vi "SEM_AMPL_RESULT.vi"(0 "Session In":refnum<visa-resource-name>="TCPIP0::K-N90X0A-00005.local::inst0::INSTR", 11 "error in":errorcluster {"code" format="%.0x"}) -> (1 "ref_freq/ref pwr":dbl[](array[numeric]), 2 "AMPL(DBC)":dbl[](array[numeric]), 3 "SPEC (DBC)":dbl[](array[numeric]), 4 "Session Out":refnum<visa-resource-name>, 15 "error out":errorcluster {"code" format="%.0x"})   [LabVIEW 2018]
doc: "Launches the Instrument I/O Assistant, which you can use to communicate with message-based instruments and graphically parse the response. For example you can communicate with an instrument that uses a serial, Ethernet, or GPIB interface."
panel:
  out "x-y":dbl
  out "Level (dBm)":dbl[](array[numeric]) format="%#.2g"
  out "LIMIT (DBC)":dbl[](array[numeric]) format="%#.2g"
  out "Margin":dbl[](array[numeric]) format="%#.2g"
  out "CA_REF_PWR":dbl
  out "CA_REF_FREQ":dbl
  out "FREQ":dbl[](array[numeric])
  in  "Timeout":u32=3000
  out "array":dbl[](array[numeric])
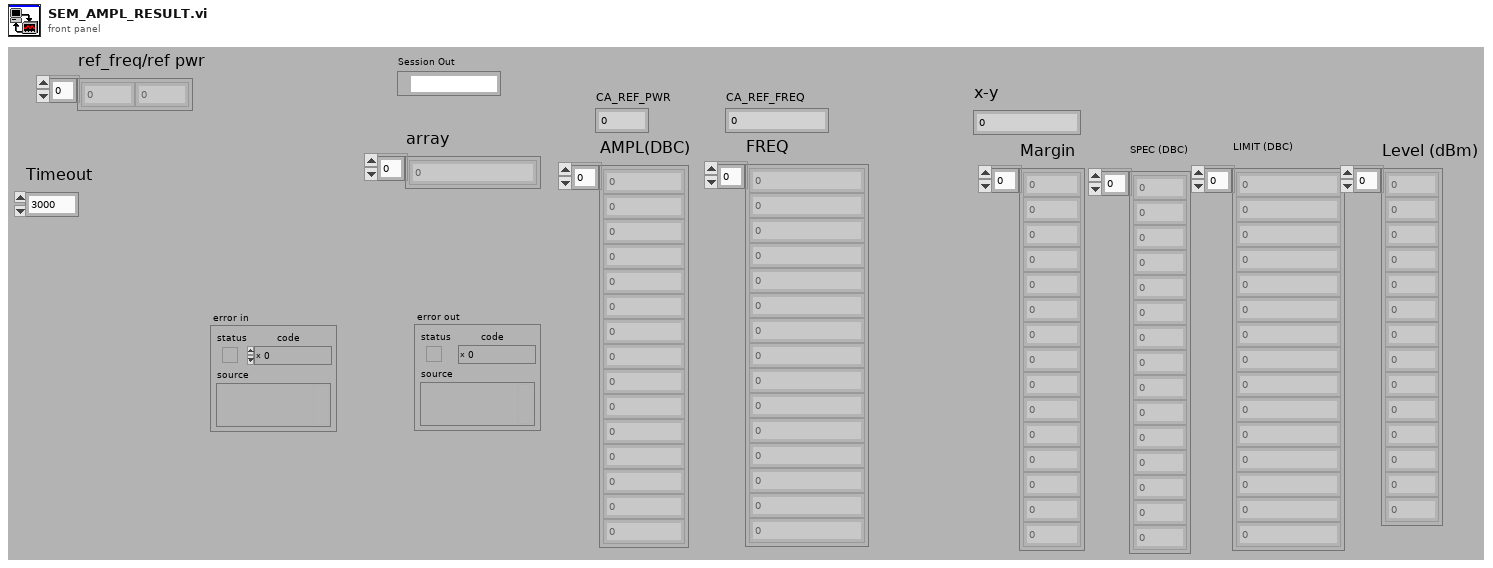
[diagram p1: front panel]
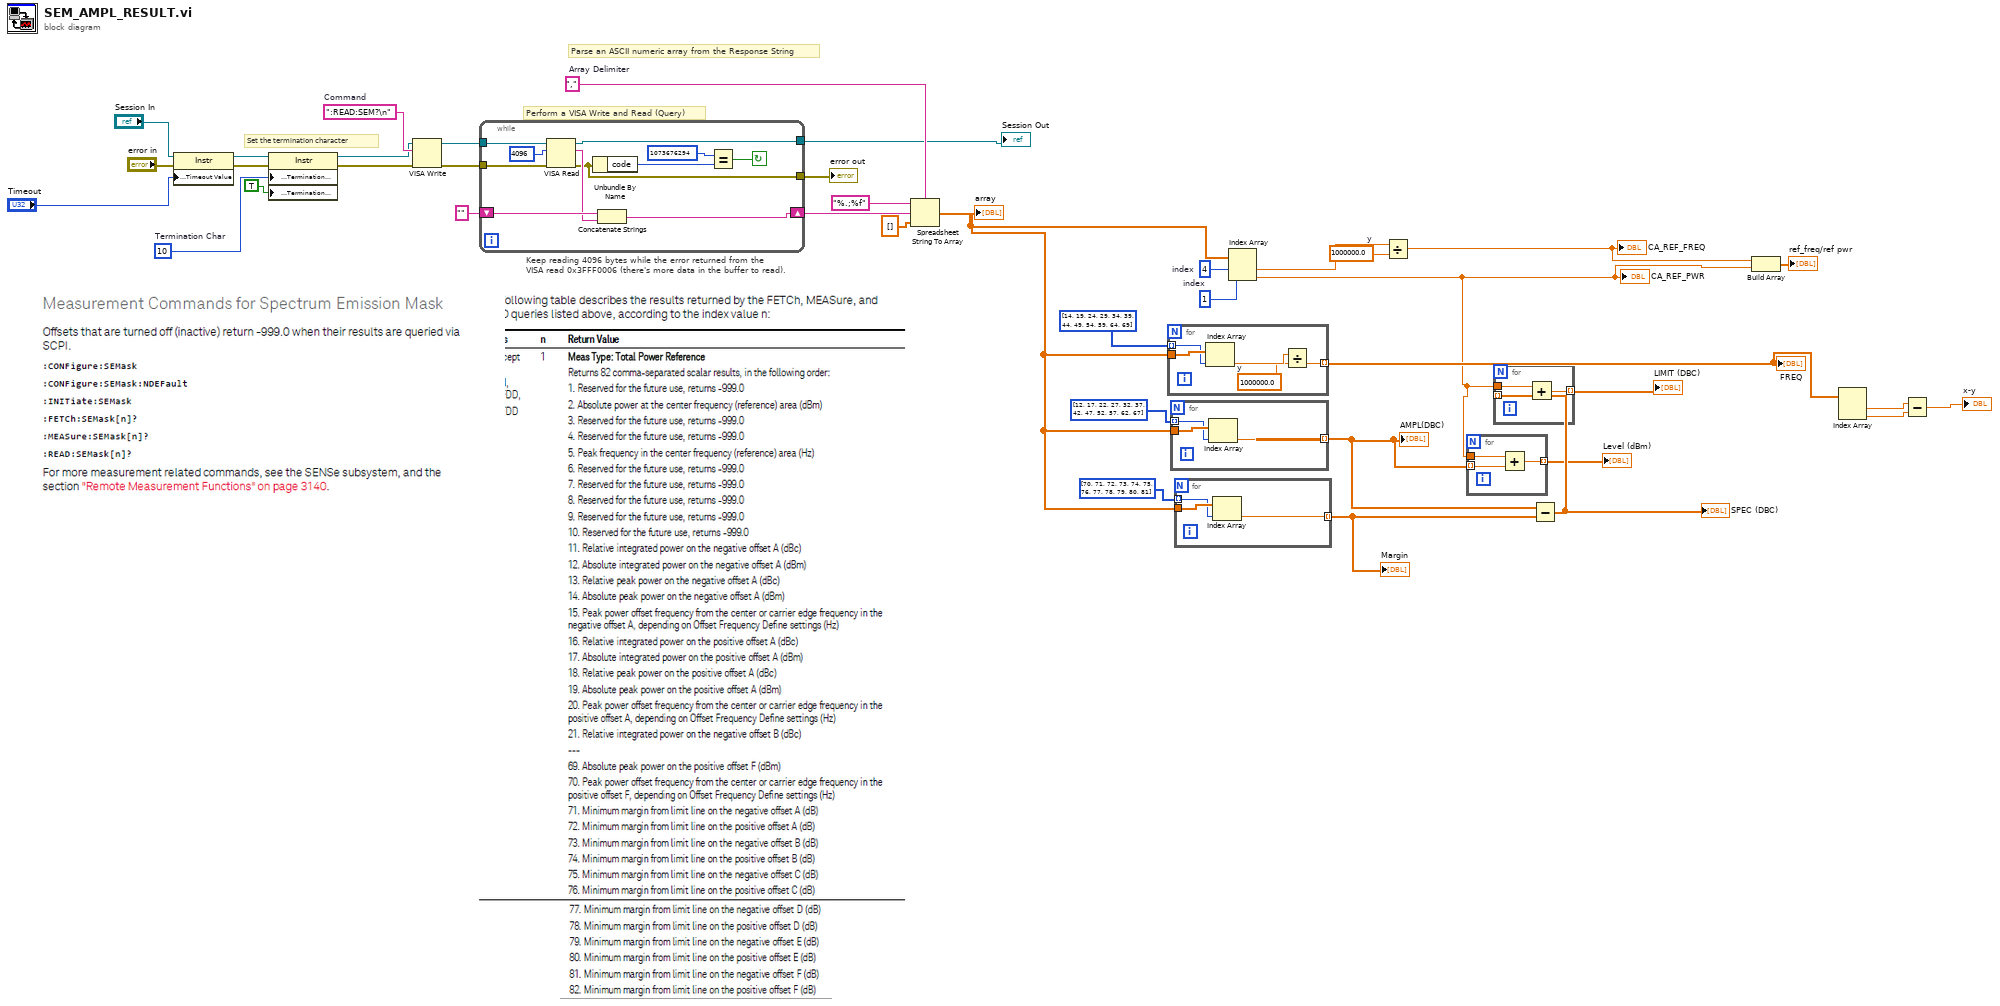
[diagram p0: block diagram]
diagram:
  w11 = 1000000.0  # y
  w19 = 1  # index
  w20 = 4  # index
  w25 = ","  # Array Delimiter
  w28 = ":READ:SEM?\n"  # Command
  w35 = u8 10  # Termination Char
  # "Parse an ASCII numeric array from the Response String"
  # "Perform a VISA Write and Read (Query)"
  # "Keep reading 4096 bytes while the error returned from the\nVISA read 0x3FFF0006 (there's more data in the buffer to read)."
  # "Set the termination character"
  n1 = property class="Instr"(reference="Session In", error in="error in", "General Settings:Timeout Value"="Timeout") -> (reference out=w34:refnum<visa-resource-name>, error out=w37:errorcluster)
  n2 = property class="Instr"(reference=w34, error in=w37, "Message Based Settings:Termination Character"=w35, "Message Based Settings:Termination Character Enable"=TRUE ("enable")) -> (reference out=w23:refnum<visa-resource-name>, error out=w36:errorcluster)
  n3 = VISA Write(VISA resource name=w23, write buffer=w28, error in (no error)=w36) -> (VISA resource name out=w32:refnum<visa-resource-name>, error out=w31:errorcluster)  [unwired: 1 out]
  n4 = while {
    tunnel: w32 -> [w47]
    shift-right: [w41] -> w24
    shift-left: "" -> [w46]
    tunnel: w31 -> [w44]
    tunnel: [w43] -> w30
    tunnel: [w40] -> w22
    stop <- w42 continue-if-true
    n5 = VISA Read(VISA resource name=w47, byte count=u32 4096 ("byte count (0)"), error in (no error)=w44) -> (VISA resource name out=w40:refnum<visa-resource-name>, read buffer=w45:string, error out=w43:errorcluster)  [unwired: 1 out]
    n6 = Unbundle By Name(w43) -> ("code"=w49:i32)
    n7 = Concatenate Strings(w46, w45) -> (w41:string)
    n8 = Equal?(x=1073676294, y=w49) -> (x = y?=w42:bool)
  }
  "error out" <- w30
  "Session Out" <- w22
  n9 = Spreadsheet String To Array(delimiter (Tab)=w25, format string="%.;%f", spreadsheet string=w24, array type (2D Dbl)=dbl[] []) -> (array=w16:dbl[])
  "array" <- w16
  n10 = for {
    tunnel: w16 -> [w55]
    tunnel: i32[] [14, 19, 24, 29, 34, 39, 44, 49, 54, 59, 64, 69] -> [w54] mode=indexing
    tunnel: [w53] -> w7 mode=indexing
    w51 = 1000000.0  # y
    n11 = Index Array(array=w55, index=w54) -> (element=w52:dbl)
    n12 = Divide(x=w52, y=w51) -> (x/y=w53:dbl)
  }
  "FREQ" <- w7
  n13 = for {
    tunnel: w16 -> [w58]
    tunnel: i32[] [12, 17, 22, 27, 32, 37, 42, 47, 52, 57, 62, 67] -> [w57] mode=indexing
    tunnel: [w56] -> w9 mode=indexing
    n14 = Index Array(array=w58, index=w57) -> (element=w56:dbl)
  }
  "AMPL(DBC)" <- w9
  n15 = for {
    tunnel: w16 -> [w61]
    tunnel: i32[] [70, 71, 72, 73, 74, 75, 76, 77, 78, 79, 80, 81] -> [w60] mode=indexing
    tunnel: [w59] -> w14 mode=indexing
    n16 = Index Array(array=w61, index=w60) -> (element=w59:dbl)
  }
  "Margin" <- w14
  n17 = Index Array(array=w16, index #1=w20, index #2=w19) -> (element #1=w12:dbl, element #2=w2:dbl)
  "CA_REF_PWR" <- w2
  n18 = Divide(x=w12, y=w11) -> (x/y=w3:dbl)
  "CA_REF_FREQ" <- w3
  n19 = for {
    tunnel: w2 -> [w64]
    tunnel: w9 -> [w63] mode=indexing
    tunnel: [w62] -> w8 mode=indexing
    n20 = Add(x=w64, y=w63) -> (x+y=w62:dbl)
  }
  "Level (dBm)" <- w8
  n21 = Subtract(x=w9, y=w14) -> (x-y=w13:dbl[])
  "SPEC (DBC)" <- w13
  n22 = for {
    tunnel: w2 -> [w67]
    tunnel: w13 -> [w66] mode=indexing
    tunnel: [w65] -> w10 mode=indexing
    n23 = Add(x=w67, y=w66) -> (x+y=w65:dbl)
  }
  "LIMIT (DBC)" <- w10
  n24 = Build Array(w3, w2) -> (→"ref_freq/ref pwr":dbl[])
  n25 = Index Array(array=w7) -> (element #1=w6:dbl, element #2=w5:dbl)  [unwired: 2 in]
  n26 = Subtract(x=w6, y=w5) -> (x-y=→"x-y":dbl)
